vi "Initialize.vi"(6 "Folder Path":path, 8 "Error In":errorcluster, 9 "Active Sequence File":refnum<k7>, 10 "Engine Reference":refnum<k7>, 11 "QPA Measurement In":refnum<class "QPA Measurement.lvclass">) -> (0 "Error Out":errorcluster, 3 "QPA Measurement out":refnum<class "QPA Measurement.lvclass">)   [LabVIEW 2016, in "QPA Measurement.lvlib" / "QPA Measurement.lvclass"]
uses:
  QPA Measurement.lvclass
  Plugins/Measurement Interface.lvlibp/Measurement Interface.lvclass
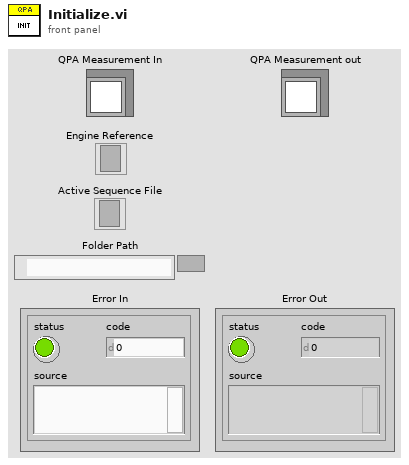
[diagram p1: front panel]
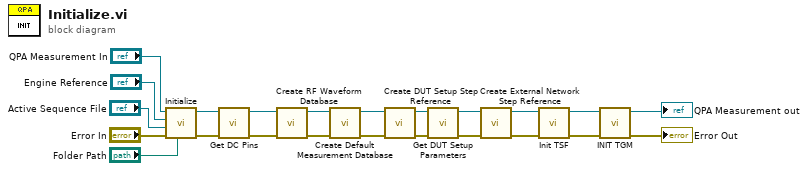
[diagram p0: block diagram]
diagram:
  n1 = call-parent "Initialize.vi"("Folder Path"="Folder Path", "Error In"="Error In", "Active Sequence File"="Active Sequence File", "Engine Reference"="Engine Reference", "Measurement Interface In"="QPA Measurement In") -> ("Error Out"=w23:errorcluster, "Measurement Interface out"=w16:refnum<class "QPA Measurement.lvclass">)  [unwired: 5 in]
  n2 = call "Get DC Pins.vi"("error in (no error)"=w23, "QPA Measurement in"=w16) -> ("error out"=w17:errorcluster, "QPA Measurement out"=w14:refnum<class "QPA Measurement.lvclass">)  [unwired: 8 in]
  n3 = call "Create RF Waveform Database.vi"("error in (no error)"=w17, "QPA Measurement in"=w14) -> ("error out"=w15:errorcluster, "QPA Measurement out"=w12:refnum<class "QPA Measurement.lvclass">)  [unwired: 8 in]
  n4 = call "Create Default Measurement Database.vi"("error in (no error)"=w15, "QPA Measurement in"=w12) -> ("error out"=w13:errorcluster, "QPA Measurement out"=w10:refnum<class "QPA Measurement.lvclass">)  [unwired: 8 in]
  n5 = call "Create DUT Setup Step Reference.vi"("error in (no error)"=w13, "QPA Measurement in"=w10) -> ("error out"=w11:errorcluster, "QPA Measurement out"=w8:refnum<class "QPA Measurement.lvclass">)  [unwired: 8 in]
  n6 = call "Get DUT Setup Parameters.vi"("error in (no error)"=w11, "QPA Measurement in"=w8) -> ("error out"=w9:errorcluster, "QPA Measurement out"=w6:refnum<class "QPA Measurement.lvclass">)  [unwired: 8 in]
  n7 = call "Create External Network Step Reference.vi"("error in (no error)"=w9, "QPA Measurement in"=w6) -> ("error out"=w7:errorcluster, "QPA Measurement out"=w4:refnum<class "QPA Measurement.lvclass">)  [unwired: 8 in]
  n8 = call "Init TSF.vi"("error in (no error)"=w7, "QPA Measurement in"=w4) -> ("error out"=w5:errorcluster, "QPA Measurement out"=w2:refnum<class "QPA Measurement.lvclass">)  [unwired: 8 in]
  n9 = call "INIT TGM.vi"("error in (no error)"=w5, "QPA Measurement in"=w2) -> ("error out"=→"Error Out":errorcluster, "QPA Measurement out"=→"QPA Measurement out":refnum<class "QPA Measurement.lvclass">)  [unwired: 8 in]
